vi "Buffer Chan Queue.vi"(8 "error in (no error)":errorcluster, 9 "BufferDurationSec":dbl, 10 "ChanDispQueue":refnum<queue>, 11 "DataProcessor in":refnum<class "DataProcessor.lvclass">) -> (0 "error out":errorcluster, 3 "DataProcessor out":refnum<class "DataProcessor.lvclass">)   [LabVIEW 2010, in "DataProcessor.lvclass"]
uses:
  DataProcessor.lvclass
  DataProcessor.lvclass/DataProcessor.ctl
panel:
  out "size(s)":i32
  out "Numeric":i32
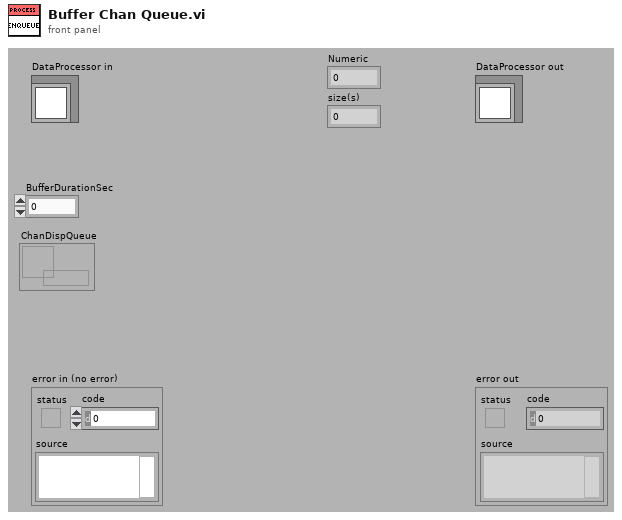
[diagram p1: front panel]
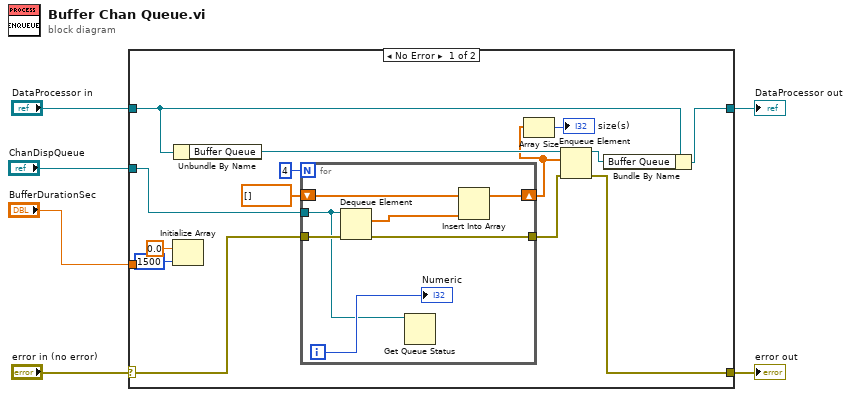
[diagram p0: block diagram]
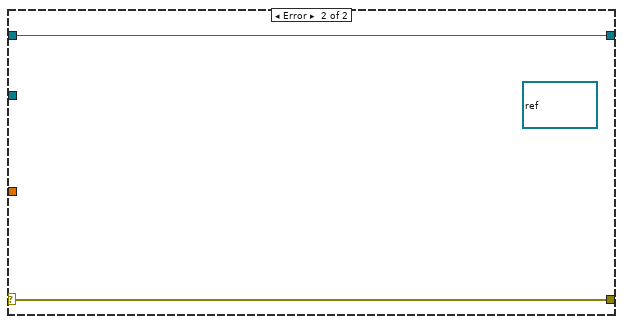
[diagram p2: hidden frame]
diagram:
  n1 = case shown="No Error" "error in (no error)" {
    selector: "error in (no error)" -> [w16 w29]
    tunnel: [w14 w29] -> w5
    tunnel: [w19 w28] -> w3
    tunnel: "DataProcessor in" -> [w20 w28]
    tunnel: "BufferDurationSec" -> [_ _]
    tunnel: "ChanDispQueue" -> [w17 _]
    frame No Error {
      n2 = Initialize Array(0.0 ("element"), 1500 ("dimension size")) -> ()  [unwired: 1 out]
      n3 = Unbundle By Name(w20) -> ("Buffer Queue"=w18:refnum<queue>)
      n4 = for {
        N: 4 -> [_]
        shift-right: [w27] -> w9
        shift-left: dbl[] [] -> [w25]
        tunnel: w17 -> [w21]
        tunnel: w16 -> [w24]
        tunnel: [w23] -> w15
        i -> [w22]
        n5 = Dequeue Element(queue=w21, error in (no error)=w24) -> (element=w26:dbl[], error out=w23:errorcluster)  [unwired: 1 in, 2 out]
        n6 = Get Queue Status(queue=w21) -> ()  [unwired: 2 in, 8 out]
        n7 = Insert Into Array(array=w25, new element=w26) -> (w27:dbl[])  [unwired: 1 in]
        "Numeric" <- w22
      }
      n8 = Array Size(array=w9) -> (size(s)=→"size(s)":i32)
      n9 = Enqueue Element(queue=w18, element=w9, error in (no error)=w15) -> (queue out=w13:refnum<queue>, error out=w14:errorcluster)  [unwired: 1 in, 1 out]
      n10 = Bundle By Name(cluster=w20, "Buffer Queue"=w13) -> (w19:refnum<class "DataProcessor.lvclass">)
    }
    frame Error {
      (unwired) refnum<queue> refnum ("Buffer Queue")
    }
  }
  "error out" <- w5
  "DataProcessor out" <- w3
